vi "Set Cursor Icon.vi"(0 "Cursor Icon":u16, 11 "error in (no error)":errorcluster) -> (15 "error out":errorcluster)   [LabVIEW 2021, in "Migrator Reusables.lvlib"]
uses:
  Migrator Reusables.lvlib
  <vilib>/Utility/cursorutil.llb/Set Cursor (Icon Pict).vi
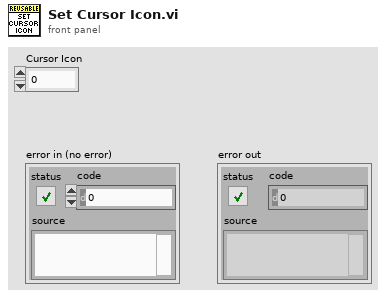
[diagram p1: front panel]
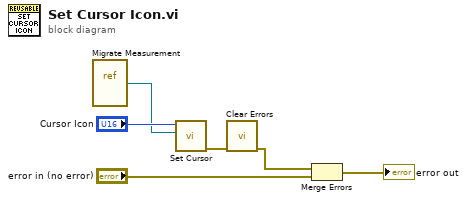
[diagram p0: block diagram]
diagram:
  n1 = vi-ref "Migrate Measurement.vi"() -> (w1:refnum<vi>)
  n2 = call-poly <vilib>:"Set Cursor.vi"("VI reference (current VI)"=w1, "icon"="Cursor Icon") -> ("error out"=w5:errorcluster)  [unwired: 8 in, 1 out]
  n3 = call <vilib>:"Clear Errors.vi"("error in (no error)"=w5) -> ("error out"=w4:errorcluster)  [unwired: 5 in, 1 out]
  n4 = Merge Errors(w4, "error in (no error)") -> (→"error out":errorcluster)
